vi "test-swerve-drve-odometry-01.vi"() -> (3 "Test Passed":bool)   [LabVIEW 2019]
uses:
  <vilib>/Rock Robotics/WPI/ThirdParty/JAS_Junk/TrajLib/SWERVE_DRIVE_ODOMETRY.ctl
  <vilib>/Rock Robotics/WPI/ThirdParty/JAS_Junk/TrajLib/POSE2D.ctl
  <vilib>/Rock Robotics/WPI/ThirdParty/JAS_Junk/TrajLib/TRANSLATION2D.ctl
  <vilib>/Rock Robotics/WPI/ThirdParty/JAS_Junk/TrajLib/ROTATION2D.ctl
  <vilib>/Rock Robotics/WPI/ThirdParty/JAS_Junk/TrajLib/SWERVE_DRIVE_KINEMATICS.ctl
  <vilib>/Analysis/Matrix/Datatypes/RealMatrix.ctl
  <vilib>/Rock Robotics/WPI/ThirdParty/JAS_Junk/TrajLib/Conv_Deg_Radians.vi
  <vilib>/Rock Robotics/WPI/ThirdParty/JAS_Junk/TrajLib/Rotation2d_CreateAngle.vi
  <vilib>/Rock Robotics/WPI/ThirdParty/JAS_Junk/TrajLib/Trajectory_Library.lvlib
  <vilib>/Analysis/Matrix/NI_Matrix.lvlib
panel:
  out "robot POSE 4":T1={"TRANSLATION"={"X"=0.0, "Y"=0.0}, "ROTATION"={"VALUE"=0.0, "COS"=1.0, "SIN"=0.0}} {"ROTATION"."SIN" format="%13.4f"; "ROTATION"."COS" format="%13.4f"; "ROTATION"."VALUE" format="%13.4f"; "TRANSLATION"."Y" format="%14.3f"; "TRANSLATION"."X" format="%14.3f"}
  out "Odom 4":T4={"POSE"={"TRANSLATION"={"X"=0.0, "Y"=0.0}, "ROTATION"={"VALUE"=0.0, "COS"=1.0, "SIN"=0.0}}, "GyroOffset"={"VALUE"=0.0, "COS"=1.0, "SIN"=0.0}, "PreviousAngle"={"VALUE"=0.0, "COS"=1.0, "SIN"=0.0}, "PrevTime"=0.0} {"PreviousAngle"."SIN" format="%13.4f"; "PreviousAngle"."COS" format="%13.4f"; "PreviousAngle"."VALUE" format="%13.4f"; "GyroOffset"."SIN" format="%13.4f"; "GyroOffset"."COS" format="%13.4f"; "GyroOffset"."VALUE" format="%13.4f"; "POSE"."ROTATION"."SIN" format="%13.4f"; "POSE"."ROTATION"."COS" format="%13.4f"; "POSE"."ROTATION"."VALUE" format="%13.4f"; "POSE"."TRANSLATION"."Y" format="%14.3f"; "POSE"."TRANSLATION"."X" format="%14.3f"}
  out "SWERVE_DRIVE_KINEMATICS":T5 {"PrevCoR"."Y" format="%14.3f"; "PrevCoR"."X" format="%14.3f"; "Modules"."Y" format="%14.3f"; "Modules"."X" format="%14.3f"}
  out "robot POSE 3":T1={"TRANSLATION"={"X"=0.0, "Y"=0.0}, "ROTATION"={"VALUE"=0.0, "COS"=1.0, "SIN"=0.0}} {"ROTATION"."SIN" format="%13.4f"; "ROTATION"."COS" format="%13.4f"; "ROTATION"."VALUE" format="%13.4f"; "TRANSLATION"."Y" format="%14.3f"; "TRANSLATION"."X" format="%14.3f"}
  out "Odom 3":T4={"POSE"={"TRANSLATION"={"X"=0.0, "Y"=0.0}, "ROTATION"={"VALUE"=0.0, "COS"=1.0, "SIN"=0.0}}, "GyroOffset"={"VALUE"=0.0, "COS"=1.0, "SIN"=0.0}, "PreviousAngle"={"VALUE"=0.0, "COS"=1.0, "SIN"=0.0}, "PrevTime"=0.0} {"PreviousAngle"."SIN" format="%13.4f"; "PreviousAngle"."COS" format="%13.4f"; "PreviousAngle"."VALUE" format="%13.4f"; "GyroOffset"."SIN" format="%13.4f"; "GyroOffset"."COS" format="%13.4f"; "GyroOffset"."VALUE" format="%13.4f"; "POSE"."ROTATION"."SIN" format="%13.4f"; "POSE"."ROTATION"."COS" format="%13.4f"; "POSE"."ROTATION"."VALUE" format="%13.4f"; "POSE"."TRANSLATION"."Y" format="%14.3f"; "POSE"."TRANSLATION"."X" format="%14.3f"}
  out "Odom 1":T4={"POSE"={"TRANSLATION"={"X"=0.0, "Y"=0.0}, "ROTATION"={"VALUE"=0.0, "COS"=1.0, "SIN"=0.0}}, "GyroOffset"={"VALUE"=0.0, "COS"=1.0, "SIN"=0.0}, "PreviousAngle"={"VALUE"=0.0, "COS"=1.0, "SIN"=0.0}, "PrevTime"=0.0} {"PreviousAngle"."SIN" format="%13.4f"; "PreviousAngle"."COS" format="%13.4f"; "PreviousAngle"."VALUE" format="%13.4f"; "GyroOffset"."SIN" format="%13.4f"; "GyroOffset"."COS" format="%13.4f"; "GyroOffset"."VALUE" format="%13.4f"; "POSE"."ROTATION"."SIN" format="%13.4f"; "POSE"."ROTATION"."COS" format="%13.4f"; "POSE"."ROTATION"."VALUE" format="%13.4f"; "POSE"."TRANSLATION"."Y" format="%14.3f"; "POSE"."TRANSLATION"."X" format="%14.3f"}
  out "Odom 0":T4={"POSE"={"TRANSLATION"={"X"=0.0, "Y"=0.0}, "ROTATION"={"VALUE"=0.0, "COS"=1.0, "SIN"=0.0}}, "GyroOffset"={"VALUE"=0.0, "COS"=1.0, "SIN"=0.0}, "PreviousAngle"={"VALUE"=0.0, "COS"=1.0, "SIN"=0.0}, "PrevTime"=0.0} {"PreviousAngle"."SIN" format="%13.4f"; "PreviousAngle"."COS" format="%13.4f"; "PreviousAngle"."VALUE" format="%13.4f"; "GyroOffset"."SIN" format="%13.4f"; "GyroOffset"."COS" format="%13.4f"; "GyroOffset"."VALUE" format="%13.4f"; "POSE"."ROTATION"."SIN" format="%13.4f"; "POSE"."ROTATION"."COS" format="%13.4f"; "POSE"."ROTATION"."VALUE" format="%13.4f"; "POSE"."TRANSLATION"."Y" format="%14.3f"; "POSE"."TRANSLATION"."X" format="%14.3f"}
  out "robot POSE 0":T1={"TRANSLATION"={"X"=0.0, "Y"=0.0}, "ROTATION"={"VALUE"=0.0, "COS"=1.0, "SIN"=0.0}} {"ROTATION"."SIN" format="%13.4f"; "ROTATION"."COS" format="%13.4f"; "ROTATION"."VALUE" format="%13.4f"; "TRANSLATION"."Y" format="%14.3f"; "TRANSLATION"."X" format="%14.3f"}
  out "robot POSE 1":T1={"TRANSLATION"={"X"=0.0, "Y"=0.0}, "ROTATION"={"VALUE"=0.0, "COS"=1.0, "SIN"=0.0}} {"ROTATION"."SIN" format="%13.4f"; "ROTATION"."COS" format="%13.4f"; "ROTATION"."VALUE" format="%13.4f"; "TRANSLATION"."Y" format="%14.3f"; "TRANSLATION"."X" format="%14.3f"}
  out "robot POSE 2":T1={"TRANSLATION"={"X"=0.0, "Y"=0.0}, "ROTATION"={"VALUE"=0.0, "COS"=1.0, "SIN"=0.0}} {"ROTATION"."SIN" format="%13.4f"; "ROTATION"."COS" format="%13.4f"; "ROTATION"."VALUE" format="%13.4f"; "TRANSLATION"."Y" format="%14.3f"; "TRANSLATION"."X" format="%14.3f"}
  out "Odom 2":T4={"POSE"={"TRANSLATION"={"X"=0.0, "Y"=0.0}, "ROTATION"={"VALUE"=0.0, "COS"=1.0, "SIN"=0.0}}, "GyroOffset"={"VALUE"=0.0, "COS"=1.0, "SIN"=0.0}, "PreviousAngle"={"VALUE"=0.0, "COS"=1.0, "SIN"=0.0}, "PrevTime"=0.0} {"PreviousAngle"."SIN" format="%13.4f"; "PreviousAngle"."COS" format="%13.4f"; "PreviousAngle"."VALUE" format="%13.4f"; "GyroOffset"."SIN" format="%13.4f"; "GyroOffset"."COS" format="%13.4f"; "GyroOffset"."VALUE" format="%13.4f"; "POSE"."ROTATION"."SIN" format="%13.4f"; "POSE"."ROTATION"."COS" format="%13.4f"; "POSE"."ROTATION"."VALUE" format="%13.4f"; "POSE"."TRANSLATION"."Y" format="%14.3f"; "POSE"."TRANSLATION"."X" format="%14.3f"}
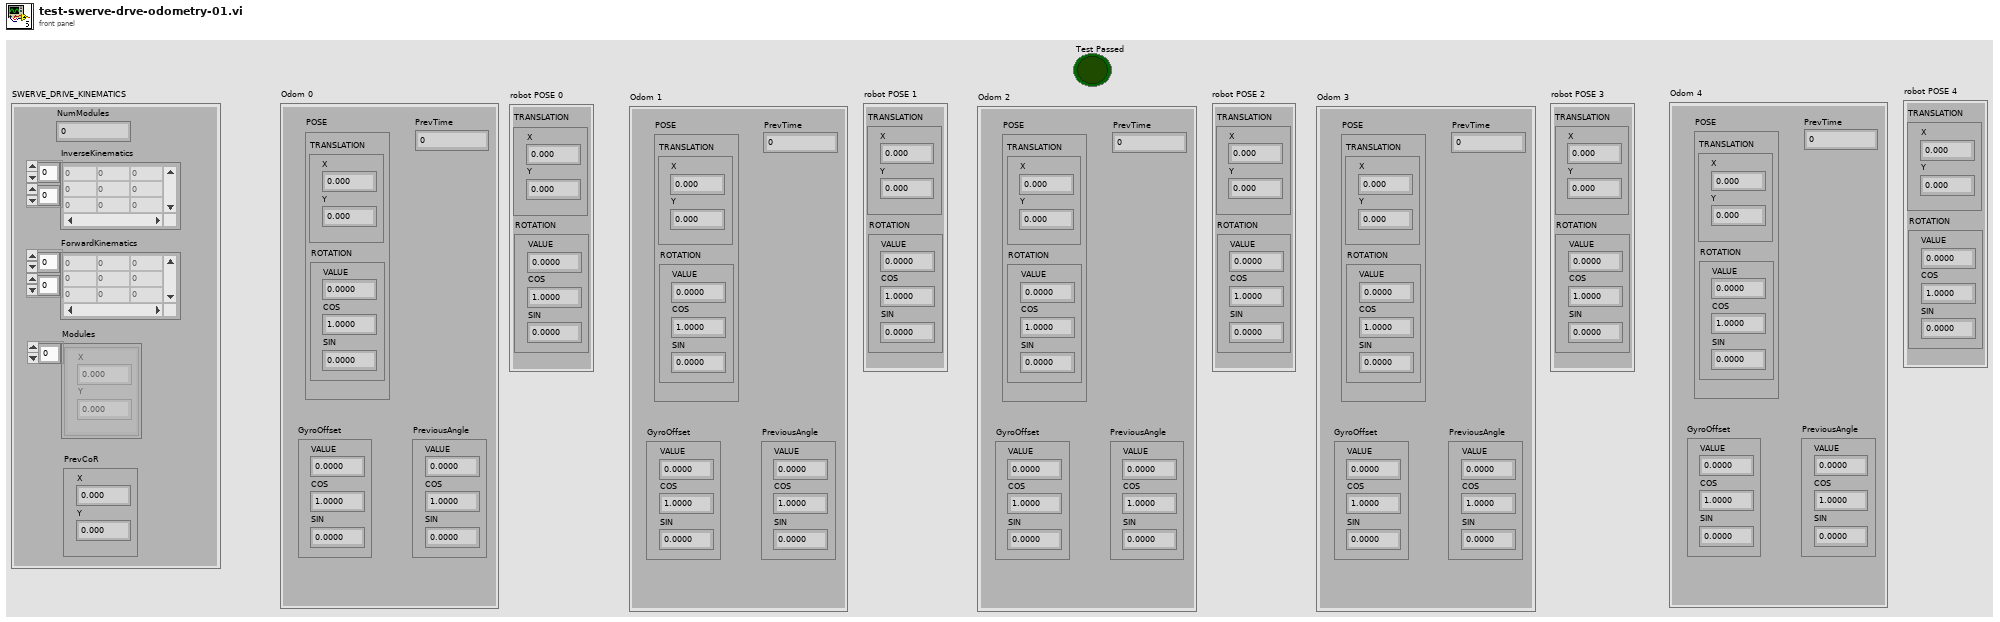
[diagram p1: front panel]
types:
  T1 = typedef "Trajectory_Library.lvlib/POSE2D.ctl" = cluster{"TRANSLATION":T2, "ROTATION":T3}
  T2 = typedef "Trajectory_Library.lvlib/TRANSLATION2D.ctl" = cluster{"X":dbl, "Y":dbl}
  T3 = typedef "Trajectory_Library.lvlib/ROTATION2D.ctl" = cluster{"VALUE":dbl, "COS":dbl, "SIN":dbl}
  T4 = typedef "Trajectory_Library.lvlib/SWERVE_DRIVE_ODOMETRY.ctl" = cluster{"POSE":T1, "GyroOffset":T3, "PreviousAngle":T3, "PrevTime":dbl}
  T5 = typedef "Trajectory_Library.lvlib/SWERVE_DRIVE_KINEMATICS.ctl" = cluster{"NumModules":i32, "InverseKinematics":T6, "ForwardKinematics":T6, "Modules":T2[], "PrevCoR":T2}
  T6 = typedef "NI_Matrix.lvlib/RealMatrix.ctl" = dbl[][]
  T7 = typedef "Trajectory_Library.lvlib/SWERVE_DRIVE_MODULE_STATE.ctl" = cluster{"Speed":dbl, "Angle":T3}
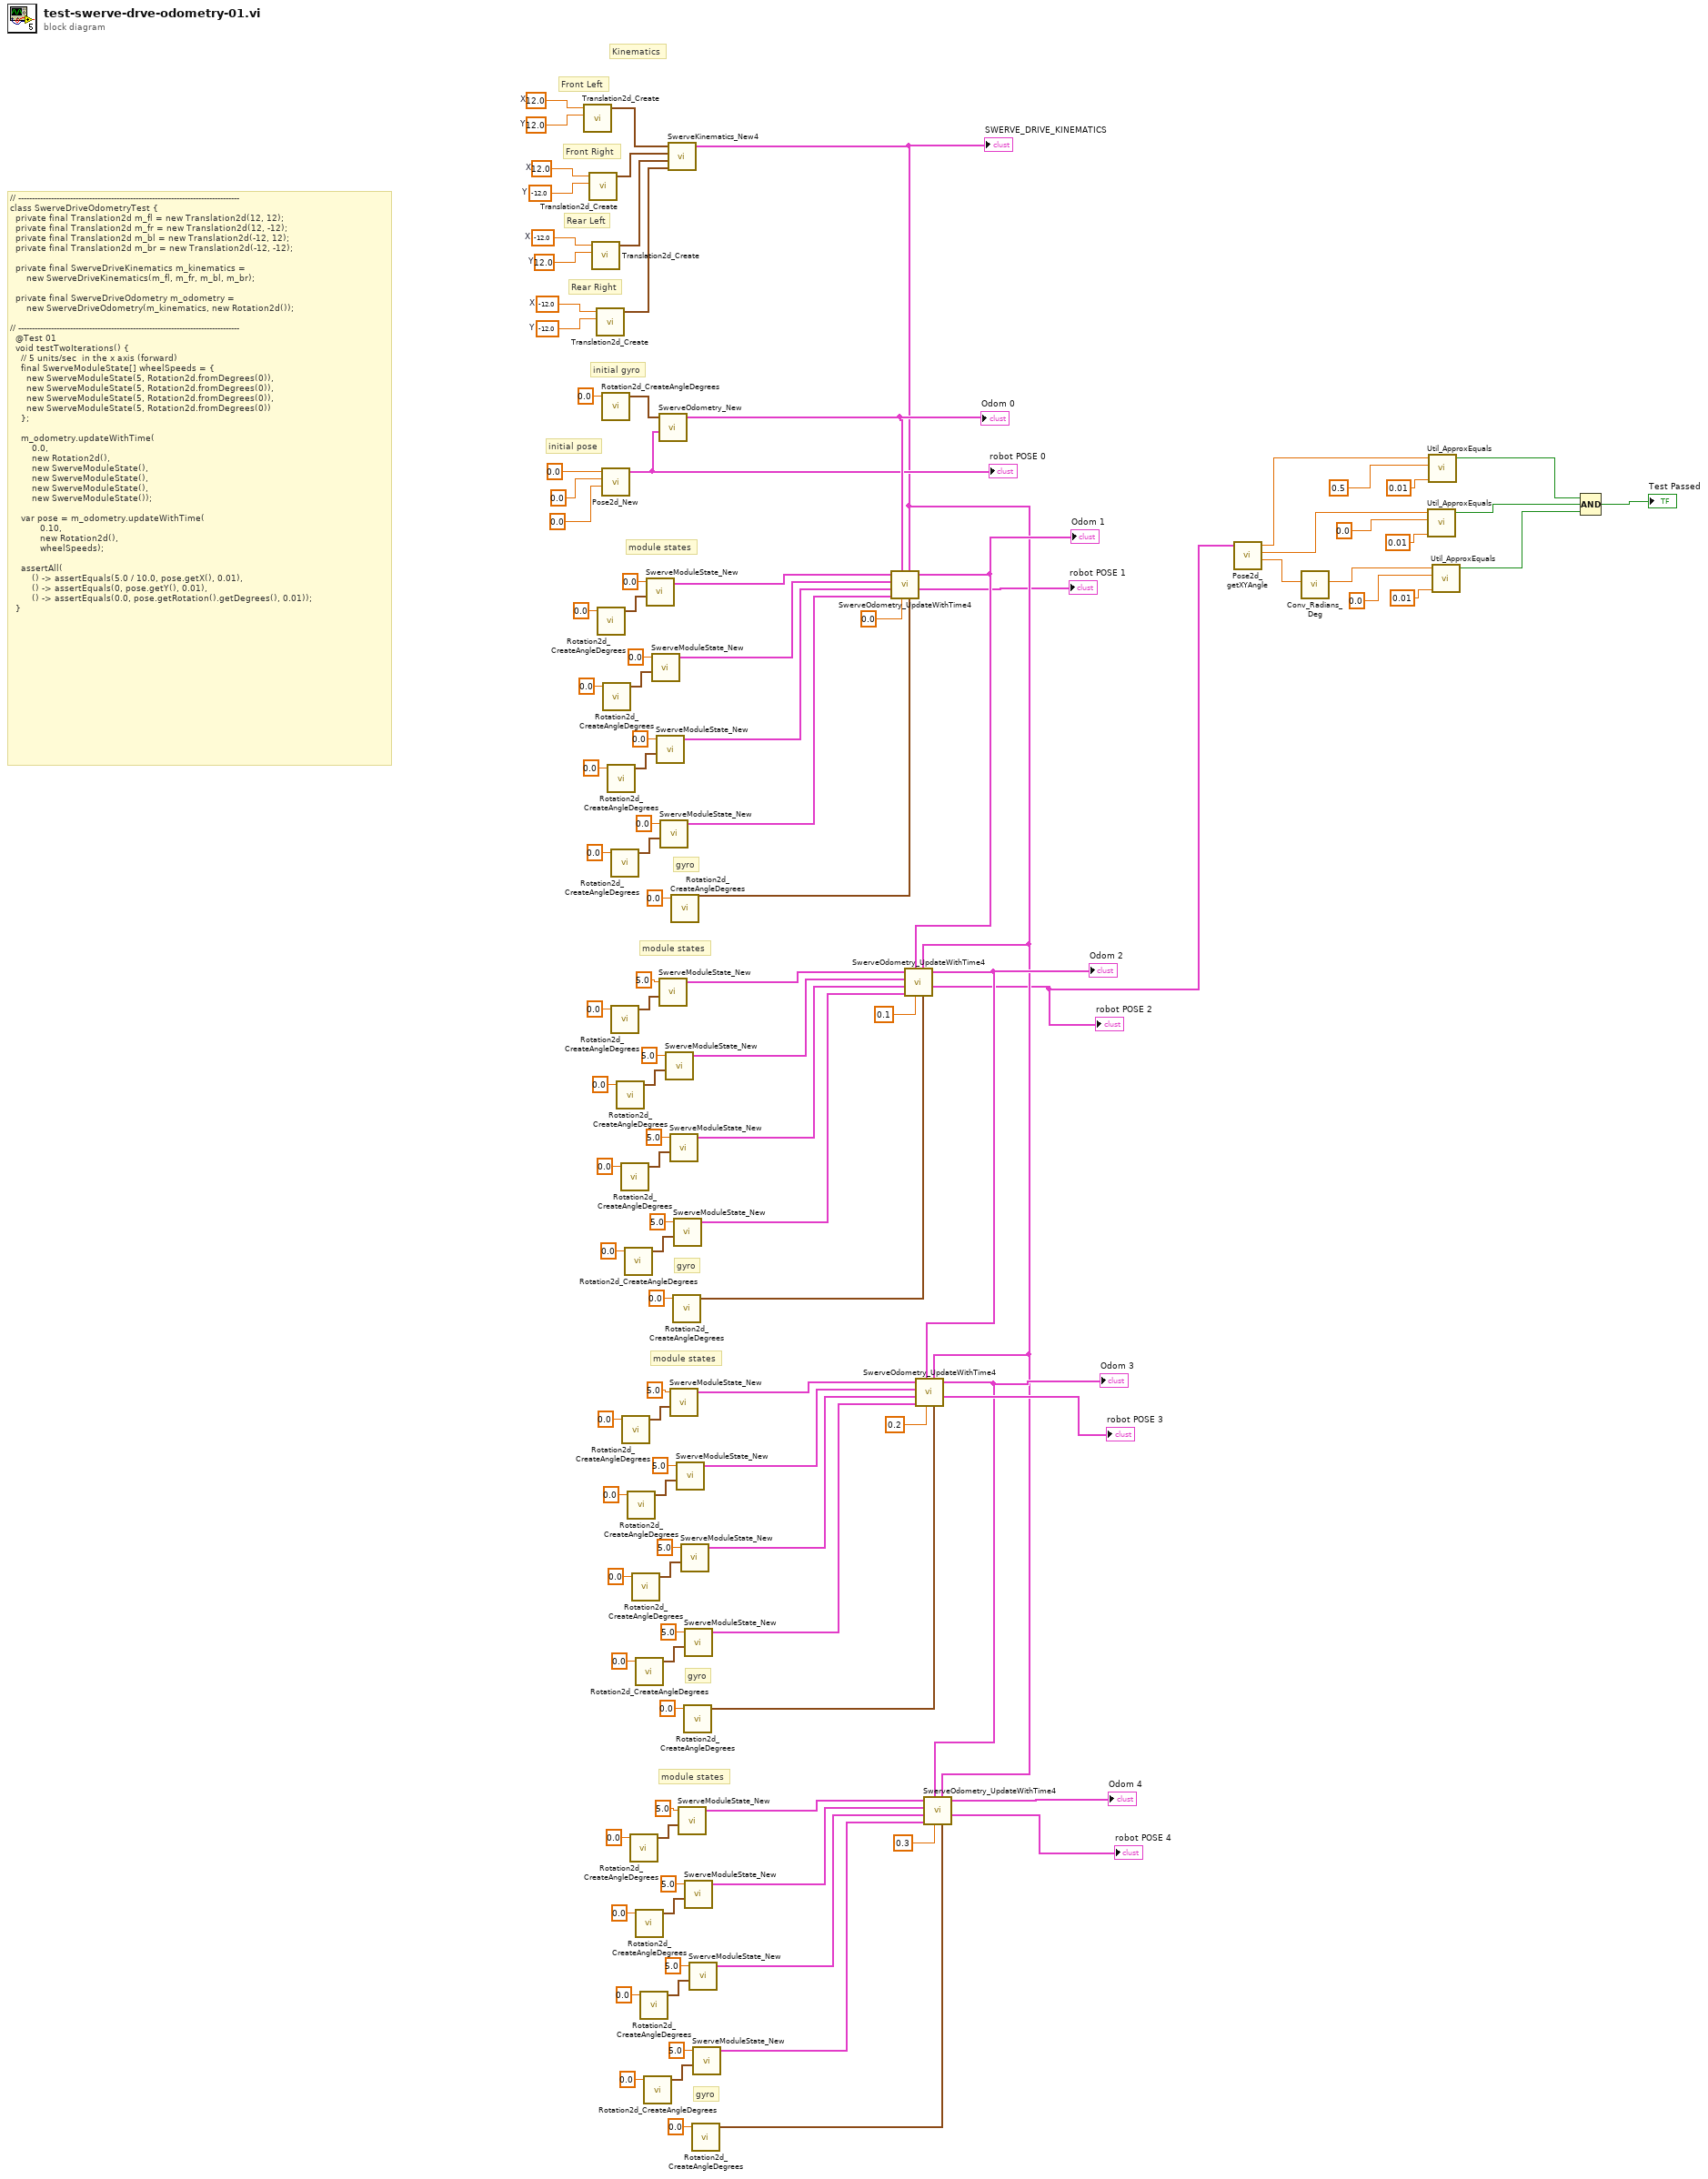
[diagram p0: block diagram]
diagram:
  w114 = -12.0  # X
  w113 = -12.0  # Y
  w112 = -12.0  # X
  w111 = 12.0  # Y
  w110 = 12.0  # X
  w109 = -12.0  # Y
  w108 = 12.0  # X
  w107 = 12.0  # Y
  # "gyro"
  # "module states"
  # "gyro"
  # "module states"
  # "initial pose"
  # "gyro"
  # "module states"
  # "gyro"
  # "module states"
  # "Kinematics"
  # "initial gyro"
  # "Rear Right"
  # "Rear Left"
  # "Front Right"
  # "Front Left"
  # "// ---------------------------------------------------------------------------------\nclass SwerveDriveOdometryTest {\n  private final Translation2d m_fl = new Translation2d(12, 12);\n  private final Translation2d m_fr = new Translation2d(12, -12);\n  private final Translation2d m_bl = new Translation2d(-12, 12);\n  private final Translation2d m_br = new Translation2d(-12, -12);\n\n  private final SwerveDriveKinematics m_kinematics =\n      new SwerveDriveKinematics(m_fl, m_fr, m_bl, m_br);\n\n  private final SwerveDriveOdometry m_odometry =\n      new SwerveDriveOdometry(m_kinematics, new Rotation2d());\n\n// ---------------------------------------------------------------------------------\n  @Test 01\n  void testTwoIterations() {\n    // 5 units/sec  in the x axis (forward)\n    final SwerveModuleState[] wheelSpeeds = {\n      new SwerveModuleState(5, Rotation2d.fromDegrees(0)),\n      new SwerveModuleState(5, Rotation2d.fromDegrees(0)),\n      new SwerveModuleState(5, Rotation2d.fromDegrees(0)),\n      new SwerveModuleState(5, Rotation2d.fromDegrees(0))\n    };\n\n    m_odometry.updateWithTime(\n        0.0,\n        new Rotation2d(),\n        new SwerveModuleState(),\n        new SwerveModuleState(),\n        new SwerveModuleState(),\n        new SwerveModuleState());\n\n    var pose = m_odometry.updateWithTime(\n           0.10, \n           new Rotation2d(), \n           wheelSpeeds);\n\n    assertAll(\n        () -> assertEquals(5.0 / 10.0, pose.getX(), 0.01),\n        () -> assertEquals(0, pose.getY(), 0.01),\n        () -> assertEquals(0.0, pose.getRotation().getDegrees(), 0.01));\n  }"
  n1 = call <vilib>:"Translation2d_Create.vi"("Y"=w107, "X"=w108) -> ("TRANSLATION"=w115:T2)  [unwired: 9 in]
  n2 = call <vilib>:"Translation2d_Create.vi"("Y"=w109, "X"=w110) -> ("TRANSLATION"=w116:T2)  [unwired: 9 in]
  n3 = call <vilib>:"Translation2d_Create.vi"("Y"=w111, "X"=w112) -> ("TRANSLATION"=w117:T2)  [unwired: 9 in]
  n4 = call <vilib>:"Translation2d_Create.vi"("Y"=w113, "X"=w114) -> ("TRANSLATION"=w118:T2)  [unwired: 9 in]
  n5 = call <vilib>:"Rotation2d_CreateAngleDegrees.vi"("Angle_Degrees"=0.0) -> ("ROTATION"=w100:T3)  [unwired: 10 in]
  n6 = call <vilib>:"Rotation2d_CreateAngleDegrees.vi"("Angle_Degrees"=0.0) -> ("ROTATION"=w103:T3)  [unwired: 10 in]
  n7 = call <vilib>:"Pose2d_New.vi"("Heading"=0.0, "Y"=0.0, "X"=0.0) -> ("out POSe"=w62:T1)  [unwired: 8 in]
  "robot POSE 0" <- w62
  n8 = call <vilib>:"Rotation2d_CreateAngleDegrees.vi"("Angle_Degrees"=0.0) -> ("ROTATION"=w97:T3)  [unwired: 10 in]
  n9 = call <vilib>:"Rotation2d_CreateAngleDegrees.vi"("Angle_Degrees"=0.0) -> ("ROTATION"=w94:T3)  [unwired: 10 in]
  n10 = call <vilib>:"Rotation2d_CreateAngleDegrees.vi"("Angle_Degrees"=0.0) -> ("ROTATION"=w91:T3)  [unwired: 10 in]
  n11 = call <vilib>:"Rotation2d_CreateAngleDegrees.vi"("Angle_Degrees"=0.0) -> ("ROTATION"=w84:T3)  [unwired: 10 in]
  n12 = call <vilib>:"Rotation2d_CreateAngleDegrees.vi"("Angle_Degrees"=0.0) -> ("ROTATION"=w81:T3)  [unwired: 10 in]
  n13 = call <vilib>:"Rotation2d_CreateAngleDegrees.vi"("Angle_Degrees"=0.0) -> ("ROTATION"=w78:T3)  [unwired: 10 in]
  n14 = call <vilib>:"Rotation2d_CreateAngleDegrees.vi"("Angle_Degrees"=0.0) -> ("ROTATION"=w59:T3)  [unwired: 10 in]
  n15 = call <vilib>:"Rotation2d_CreateAngleDegrees.vi"("Angle_Degrees"=0.0) -> ("ROTATION"=w75:T3)  [unwired: 10 in]
  n16 = call <vilib>:"Rotation2d_CreateAngleDegrees.vi"("Angle_Degrees"=0.0) -> ("ROTATION"=w56:T3)  [unwired: 10 in]
  n17 = call <vilib>:"Rotation2d_CreateAngleDegrees.vi"("Angle_Degrees"=0.0) -> ("ROTATION"=w38:T3)  [unwired: 10 in]
  n18 = call <vilib>:"Rotation2d_CreateAngleDegrees.vi"("Angle_Degrees"=0.0) -> ("ROTATION"=w53:T3)  [unwired: 10 in]
  n19 = call <vilib>:"Rotation2d_CreateAngleDegrees.vi"("Angle_Degrees"=0.0) -> ("ROTATION"=w50:T3)  [unwired: 10 in]
  n20 = call <vilib>:"Rotation2d_CreateAngleDegrees.vi"("Angle_Degrees"=0.0) -> ("ROTATION"=w35:T3)  [unwired: 10 in]
  n21 = call <vilib>:"Rotation2d_CreateAngleDegrees.vi"("Angle_Degrees"=0.0) -> ("ROTATION"=w32:T3)  [unwired: 10 in]
  n22 = call <vilib>:"Rotation2d_CreateAngleDegrees.vi"("Angle_Degrees"=0.0) -> ("ROTATION"=w29:T3)  [unwired: 10 in]
  n23 = call <vilib>:"SwerveModuleState_New.vi"("ROTATION"=w100, "Speed"=0.0) -> ("SWERVE_DRIVE_MODULE_STATE"=w89:T7)  [unwired: 9 in]
  n24 = call <vilib>:"SwerveModuleState_New.vi"("ROTATION"=w97, "Speed"=0.0) -> ("SWERVE_DRIVE_MODULE_STATE"=w88:T7)  [unwired: 9 in]
  n25 = call <vilib>:"SwerveModuleState_New.vi"("ROTATION"=w94, "Speed"=0.0) -> ("SWERVE_DRIVE_MODULE_STATE"=w87:T7)  [unwired: 9 in]
  n26 = call <vilib>:"SwerveOdometry_New.vi"("InitialPose"=w62, "gyroAngle"=w103) -> ("SWERVE_DRIVE_ODOMETRY"=w63:T4)  [unwired: 9 in]
  "Odom 0" <- w63
  n27 = call <vilib>:"SwerveModuleState_New.vi"("ROTATION"=w84, "Speed"=5.0) -> ("SWERVE_DRIVE_MODULE_STATE"=w73:T7)  [unwired: 9 in]
  n28 = call <vilib>:"SwerveModuleState_New.vi"("ROTATION"=w91, "Speed"=0.0) -> ("SWERVE_DRIVE_MODULE_STATE"=w86:T7)  [unwired: 9 in]
  n29 = call <vilib>:"SwerveModuleState_New.vi"("ROTATION"=w81, "Speed"=5.0) -> ("SWERVE_DRIVE_MODULE_STATE"=w72:T7)  [unwired: 9 in]
  n30 = call <vilib>:"SwerveKinematics_New4.vi"("wheel 3"=w118, "wheel 2"=w117, "wheel 1"=w116, "wheel 0"=w115) -> ("SWERVE_DRIVE_KINEMATICS"=w17:T5)  [unwired: 7 in]
  "SWERVE_DRIVE_KINEMATICS" <- w17
  n31 = call <vilib>:"SwerveModuleState_New.vi"("ROTATION"=w78, "Speed"=5.0) -> ("SWERVE_DRIVE_MODULE_STATE"=w71:T7)  [unwired: 9 in]
  n32 = call <vilib>:"SwerveModuleState_New.vi"("ROTATION"=w59, "Speed"=5.0) -> ("SWERVE_DRIVE_MODULE_STATE"=w48:T7)  [unwired: 9 in]
  n33 = call <vilib>:"Rotation2d_CreateAngleDegrees.vi"("Angle_Degrees"=0.0) -> ("ROTATION"=w68:T3)  [unwired: 10 in]
  n34 = call <vilib>:"Rotation2d_CreateAngleDegrees.vi"("Angle_Degrees"=0.0) -> ("ROTATION"=w64:T3)  [unwired: 10 in]
  n35 = call <vilib>:"SwerveModuleState_New.vi"("ROTATION"=w75, "Speed"=5.0) -> ("SWERVE_DRIVE_MODULE_STATE"=w70:T7)  [unwired: 9 in]
  n36 = call <vilib>:"SwerveModuleState_New.vi"("ROTATION"=w56, "Speed"=5.0) -> ("SWERVE_DRIVE_MODULE_STATE"=w47:T7)  [unwired: 9 in]
  n37 = call <vilib>:"SwerveModuleState_New.vi"("ROTATION"=w38, "Speed"=5.0) -> ("SWERVE_DRIVE_MODULE_STATE"=w27:T7)  [unwired: 9 in]
  n38 = call <vilib>:"SwerveModuleState_New.vi"("ROTATION"=w53, "Speed"=5.0) -> ("SWERVE_DRIVE_MODULE_STATE"=w46:T7)  [unwired: 9 in]
  n39 = call <vilib>:"Rotation2d_CreateAngleDegrees.vi"("Angle_Degrees"=0.0) -> ("ROTATION"=w42:T3)  [unwired: 10 in]
  n40 = call <vilib>:"SwerveModuleState_New.vi"("ROTATION"=w50, "Speed"=5.0) -> ("SWERVE_DRIVE_MODULE_STATE"=w45:T7)  [unwired: 9 in]
  n41 = call <vilib>:"SwerveModuleState_New.vi"("ROTATION"=w35, "Speed"=5.0) -> ("SWERVE_DRIVE_MODULE_STATE"=w26:T7)  [unwired: 9 in]
  n42 = call <vilib>:"SwerveModuleState_New.vi"("ROTATION"=w32, "Speed"=5.0) -> ("SWERVE_DRIVE_MODULE_STATE"=w25:T7)  [unwired: 9 in]
  n43 = call <vilib>:"Rotation2d_CreateAngleDegrees.vi"("Angle_Degrees"=0.0) -> ("ROTATION"=w21:T3)  [unwired: 10 in]
  n44 = call <vilib>:"SwerveModuleState_New.vi"("ROTATION"=w29, "Speed"=5.0) -> ("SWERVE_DRIVE_MODULE_STATE"=w24:T7)  [unwired: 9 in]
  n45 = call <vilib>:"SwerveOdometry_UpdateWithTime4.vi"("gyroAngle"=w68, "SWERVE_DRIVE_KINEMATICS"=w17, "Time"=0.0, "in SWERVE_DRIVE_ODOMETRY"=w63, "Wheel State 3"=w86, "Wheel State 2"=w87, "Wheel State 1"=w88, "Wheel State 0"=w89) -> ("robot POSE"=→"robot POSE 1":T1, "out SWERVE_DRIVE_ODOMETRY"=w61:T4)  [unwired: 2 in]
  "Odom 1" <- w61
  n46 = call <vilib>:"SwerveOdometry_UpdateWithTime4.vi"("gyroAngle"=w64, "SWERVE_DRIVE_KINEMATICS"=w17, "Time"=0.1, "in SWERVE_DRIVE_ODOMETRY"=w61, "Wheel State 3"=w70, "Wheel State 2"=w71, "Wheel State 1"=w72, "Wheel State 0"=w73) -> ("robot POSE"=w1:T1, "out SWERVE_DRIVE_ODOMETRY"=w40:T4)  [unwired: 2 in]
  "Odom 2" <- w40
  "robot POSE 2" <- w1
  n47 = call <vilib>:"SwerveOdometry_UpdateWithTime4.vi"("gyroAngle"=w42, "SWERVE_DRIVE_KINEMATICS"=w17, "Time"=0.2, "in SWERVE_DRIVE_ODOMETRY"=w40, "Wheel State 3"=w45, "Wheel State 2"=w46, "Wheel State 1"=w47, "Wheel State 0"=w48) -> ("robot POSE"=→"robot POSE 3":T1, "out SWERVE_DRIVE_ODOMETRY"=w18:T4)  [unwired: 2 in]
  "Odom 3" <- w18
  n48 = call <vilib>:"SwerveOdometry_UpdateWithTime4.vi"("gyroAngle"=w21, "SWERVE_DRIVE_KINEMATICS"=w17, "Time"=0.3, "in SWERVE_DRIVE_ODOMETRY"=w18, "Wheel State 3"=w24, "Wheel State 2"=w25, "Wheel State 1"=w26, "Wheel State 0"=w27) -> ("robot POSE"=→"robot POSE 4":T1, "out SWERVE_DRIVE_ODOMETRY"=→"Odom 4":T4)  [unwired: 2 in]
  n49 = call <vilib>:"Pose2d_getXYAngle.vi"("in POSE"=w1) -> ("Angle"=w13:dbl, "Y"=w10:dbl, "X"=w11:dbl)  [unwired: 8 in]
  n50 = call <vilib>:"Conv_Radians_Deg.vi"("Radians"=w13) -> ("Degrees"=w9:dbl)  [unwired: 10 in]
  n51 = call <vilib>:"Util_ApproxEquals.vi"("Tolerance"=0.01, "Value 2"=0.0, "Value 1"=w10) -> ("ApproxEquals"=w4:bool)  [unwired: 8 in]
  n52 = call <vilib>:"Util_ApproxEquals.vi"("Tolerance"=0.01, "Value 2"=0.5, "Value 1"=w11) -> ("ApproxEquals"=w5:bool)  [unwired: 8 in]
  n53 = call <vilib>:"Util_ApproxEquals.vi"("Tolerance"=0.01, "Value 2"=0.0, "Value 1"=w9) -> ("ApproxEquals"=w3:bool)  [unwired: 8 in]
  n54 = Compound Arithmetic op=AND(w5, w4, w3) -> (→"Test Passed":bool)
